vi "Notify Subscribers.vi"(8 "error in (no error)":errorcluster, 10 "PublishRequest":refnum<class "PublishRequest.lvclass">, 11 "Topic in":refnum<class "Topic.lvclass">) -> (0 "error out":errorcluster, 3 "Topic out":refnum<class "Topic.lvclass">)   [LabVIEW 2017, in "Mediator.lvlib" / "Topic.lvclass"]
doc: "<License>\nCopyright © 2017 Composed Systems, LLC | All rights reserved\nwww.composed.io\n\nAuthor: Ethan Stern <ethan.stern@composed.io>\n\nThis software is provided \"AS IS\" WITHOUT WARRANTIES, either express or implied, AND IS FOR EDUCATIONAL PURPOSES ONLY.\n</License>"
uses:
  <vilib>/gpm_packages/@cs/mva-core/Source/Mediator/Topic/Topic.lvclass
  <vilib>/gpm_packages/@cs/mva-core/Source/IMediator/PublishRequest/PublishRequest.lvclass
  <vilib>/gpm_packages/@cs/mva-core/Source/Mediator/Topic/Topic.lvclass/Topic.ctl
  <vilib>/gpm_packages/@cs/mva-core/Source/IMediator/PublishRequest/PublishRequest.lvclass/PublishRequest.ctl
  <vilib>/gpm_packages/@cs/mva-core/Source/IMediator/ISubscriptionPolicy/ISubscriptionPolicy.lvclass/ISubscriptionPolicy.ctl
  <vilib>/gpm_packages/@cs/mva-core/Source/IMediator/ISubscriptionPolicy/Execute Subscription Policy.vi
  <vilib>/gpm_packages/@cs/mva-core/Source/IMediator/ISubscriptionPolicy/ISubscriptionPolicy.lvclass
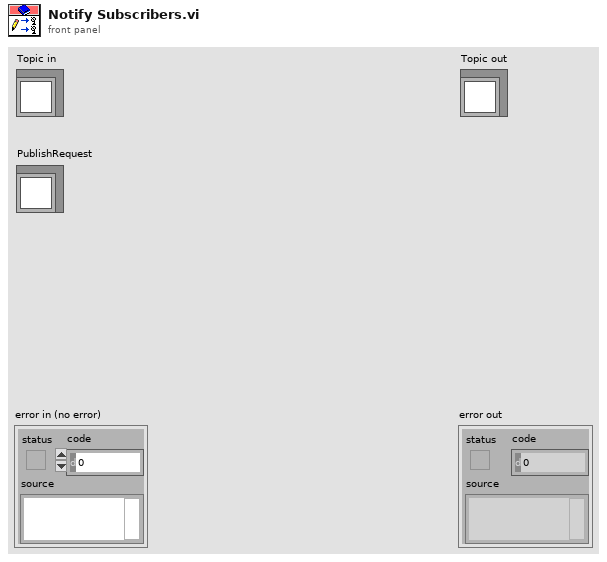
[diagram p1: front panel]
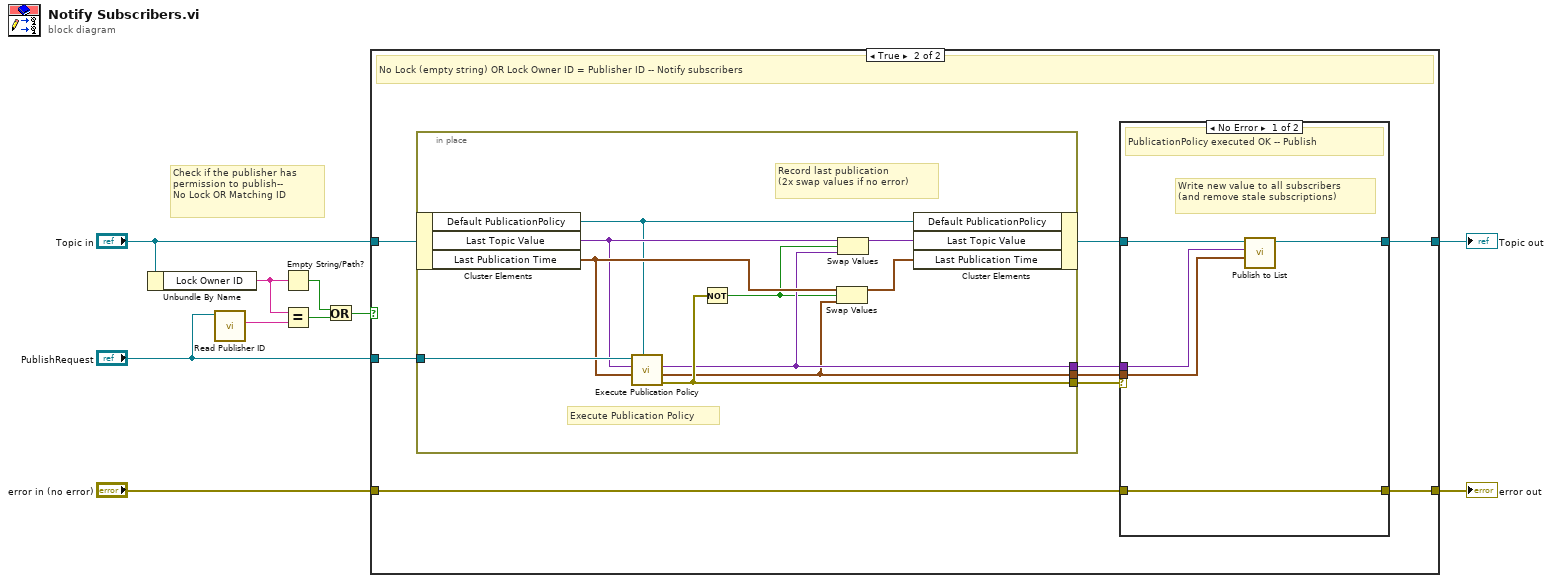
[diagram p0: block diagram]
diagram:
  # "Check if the publisher has\npermission to publish--\nNo Lock OR Matching ID"
  n1 = Unbundle By Name("Topic in") -> ("Lock Owner ID"=w6:string)
  n2 = call <vilib>:"Read Publisher ID.vi"("PublishRequest In"="PublishRequest") -> ("Publisher ID"=w1:string)  [unwired: 10 in]
  n3 = Empty String/Path?(string/path=w6) -> (empty?=w5:bool)
  n4 = Equal?(x=w6, y=w1) -> (x = y?=w4:bool)
  n5 = Or(x=w5, y=w4) -> (x .or. y?=w3:bool)
  n6 = case shown="True" w3 {
    tunnel: "error in (no error)" -> [w12 w21]
    tunnel: [w12 w20] -> w9
    tunnel: [w11 w19] -> w8
    tunnel: "Topic in" -> [w11 w14]
    tunnel: "PublishRequest" -> [_ w18]
    frame False {
      # "This publication was not from the lock holder -- Ignore it"
    }
    frame True {
      # "No Lock (empty string) OR Lock Owner ID = Publisher ID -- Notify subscribers"
      n7 = in-place {
        in-place-border: w18 -> [w31]
        in-place-border: [w24] -> w17
        in-place-border: [w27] -> w16
        in-place-border: [w22] -> w15
        # "Record last publication\n(2x swap values if no error)"
        # "Execute Publication Policy"
        n8 = in-place-cluster #1(w14) -> ("Default PublicationPolicy"=w25:refnum<class "IPublicationPolicy.lvclass">, "Last Topic Value"=w26:variant, "Last Publication Time"=w29:timestamp)
        n9 = call-dynamic "Execute Publication Policy.vi"("Default PublicationPolicy"=w25, "Last Publish Time"=w29, "Last Published Value"=w26, "PublishRequest"=w31) -> ("error out (Reject Publication)"=w27:errorcluster, "Publication Time"=w22:timestamp, "Value to Publish"=w24:variant)  [unwired: 5 in]
        n10 = Not(x=w27) -> (.not. x?=w23:bool)
        n11 = Swap Values(12:w29, 13:w23, 14:w22) -> (1:w28:timestamp)  [unwired: 1 out]
        n12 = Swap Values(12:w26, 13:w23, 14:w24) -> (1:w30:variant)  [unwired: 1 out]
        n13 = in-place-cluster #1("Default PublicationPolicy"=w25, "Last Topic Value"=w30, "Last Publication Time"=w28) -> (w13:refnum<class "Topic.lvclass">)
      }
      n14 = case shown="No Error" w16 {
        tunnel: w21 -> [w36 w38]
        tunnel: [w36 w38] -> w20
        tunnel: [w35 w37] -> w19
        tunnel: w13 -> [w34 w37]
        tunnel: w17 -> [w32 _]
        tunnel: w15 -> [w33 _]
        frame No Error {
          # "Write new value to all subscribers\n(and remove stale subscriptions)"
          # "PublicationPolicy executed OK -- Publish"
          n15 = call <vilib>:"Publish to List.vi"("Publication Time"=w33, "Value to Publish"=w32, "Topic in"=w34) -> ("Topic out"=w35:refnum<class "Topic.lvclass">)  [unwired: 8 in]
        }
        frame Error {
          # "Error executing PublicationPolicy -- Do not publish"
        }
      }
    }
  }
  "error out" <- w9
  "Topic out" <- w8
